vi "Write To Log.vi"(9 "log level":T1, 10 "message":string, 11 "connection in":refnum<class "Low Level Connection.lvclass">) -> (3 "connection out":refnum<class "Low Level Connection.lvclass">)   [LabVIEW 2020, in "NI_SFTP.lvlib" / "Low Level Connection.lvclass"]
uses:
  <vilib>/net/SFTP/Low Level Connection/Low Level Connection.lvclass
  <vilib>/net/SFTP/Low Level Connection/Log Level.ctl
  <vilib>/net/SFTP/Low Level Connection/Low Level Connection.lvclass/Low Level Connection.ctl
  <vilib>/Utility/Debug Log/Debug Log.lvlib
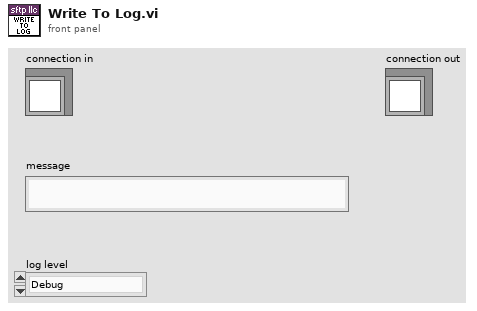
[diagram p1: front panel]
types:
  T1 = typedef "NI_SFTP.lvlib/Low Level Connection.lvclass/Log Level.ctl" = enum16{"Debug", "Information", "Warning", "Error", "None"}
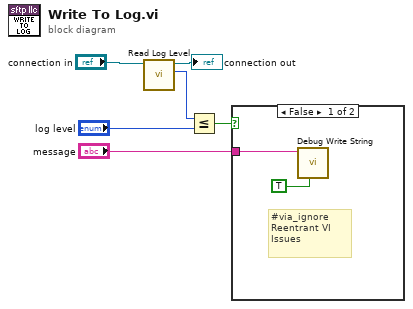
[diagram p0: block diagram]
diagram:
  n1 = call <vilib>:"Read Log Level.vi"("connection in"="connection in") -> ("log level"=w3:T1, "connection out"=→"connection out":refnum<class "Low Level Connection.lvclass">)  [unwired: 9 in]
  n2 = Less Or Equal?(x=w3, y="log level") -> (x <= y?=w2:bool)
  n3 = case shown="False" w2 {
    tunnel: "message" -> [w8 _]
    frame False {
      # "#via_ignore Reentrant VI Issues"
      n4 = call <vilib>:"Debug Write String.vi"("include timestamp? (F)"=TRUE, "value"=w8) -> ()  [unwired: 9 in, 1 out]
    }
    frame True {
    }
  }
